vi "Self-Test.vi"(8 "error in (no error)":errorcluster, 11 "VISA resource name":refnum<visa-resource-name>) -> (0 "error out":errorcluster, 1 "Self-Test Result Message":string, 2 "Self-Test Result Code":i32, 3 "VISA resource name out":refnum<visa-resource-name>)   [LabVIEW 2012, in "Temptronic TP04300.lvlib"]
doc: "Runs the instrument's self-test routine and returns the test results."
uses:
  <instrlib>/Temptronic TP04300/Temptronic TP04300.lvlib
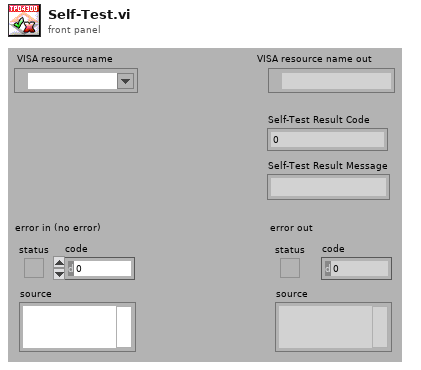
[diagram p1: front panel]
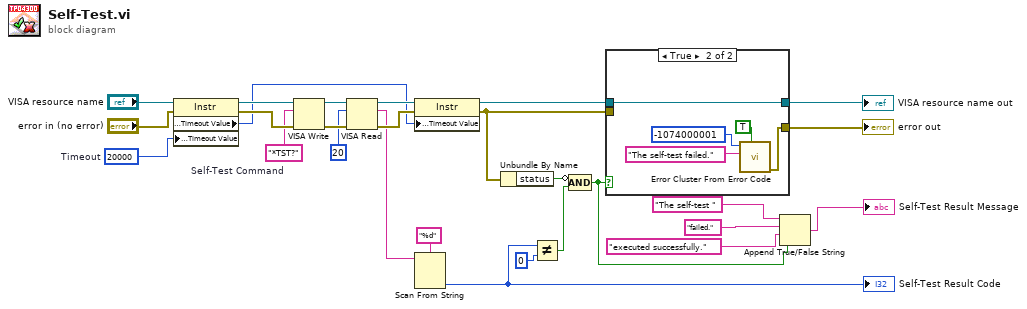
[diagram p0: block diagram]
diagram:
  w18 = u32 20000  # Timeout
  w14 = "*TST?"  # Self-Test Command
  n1 = property class="Instr"(reference="VISA resource name", error in="error in (no error)", "General Settings:Timeout Value"=w18) -> (reference out=w16:refnum<visa-resource-name>, error out=w17:errorcluster, "General Settings:Timeout Value"=w15:u32)
  n2 = VISA Write(VISA resource name=w16, write buffer=w14, error in (no error)=w17) -> (VISA resource name out=w24:refnum<visa-resource-name>, error out=w23:errorcluster)  [unwired: 1 out]
  n3 = VISA Read(VISA resource name=w24, byte count=u32 20 ("byte count (20)"), error in (no error)=w23) -> (VISA resource name out=w26:refnum<visa-resource-name>, read buffer=w19:string, error out=w25:errorcluster)  [unwired: 1 out]
  n4 = property class="Instr"(reference=w26, error in=w25, "General Settings:Timeout Value"=w15) -> (reference out=w13:refnum<visa-resource-name>, error out=w12:errorcluster)
  n5 = Scan From String(format string="%d", input string=w19) -> (output 1=w9:i32)  [unwired: 3 in, 3 out]
  "Self-Test Result Code" <- w9
  n6 = Unbundle By Name(w12) -> ("status"=w10:bool)
  n7 = Not Equal?(x=w9, y=0) -> (x != y?=w11:bool)
  n8 = Compound Arithmetic op=AND(invert w10, w11) -> (w3:bool)
  n9 = case shown="True" w3 {
    tunnel: w13 -> [w29 w34]
    tunnel: w12 -> [w28 _]
    tunnel: [w28 w30] -> w1
    tunnel: [w29 w34] -> w2
    frame False {
    }
    frame True {
      n10 = call <vilib>:"Error Cluster From Error Code.vi"("show call chain? (False)"=TRUE, "error message (\"\")"="The self-test failed." ("Source (VI Name)"), "error code (0)"=-1074000001 ("Code")) -> ("error out"=w30:errorcluster)  [unwired: 6 in]
    }
  }
  "VISA resource name out" <- w2
  "error out" <- w1
  n11 = Append True/False String(1:w3, 2:"executed successfully." ("Format String"), 3:"failed." ("Source (VI Name)"), 4:"The self-test " ("Source (VI Name)")) -> (0:→"Self-Test Result Message":string)
